vi "Find Exact Peak.vi"(0 "window":T1(ring)=enum."7 Term B-Harris", 1 "Freq. Resolution":dbl=1e-08 format="%0.2e", 2 "Size of FFT (N)":i32=1024 min=0 step=1, 3 "A0":dbl=3.738613052908998e-10 format="%0.8f", 4 "A1":dbl=3.686220325397741e-10 format="%0.8f") -> (5 "A exact":dbl=3.926212591970866e-10 format="%0.8f", 6 "f exact":dbl format="%0.8f")   [LabVIEW 2017, in "NI_AALPro.lvlib"]
doc: "Finds an accurate approximation to the peak response and frequency location using the window coefficients and a binary search algorithm. The best guess is initialized to the center of the frequency bins and is moved within the search loop until the window responses at the bin edges closely approximate the observed magnitude responses of the original spectrum."
uses:
  <vilib>/Analysis/NI_AALPro.lvlib
panel:
  in  "max iterations":i32=100 min=0 step=1
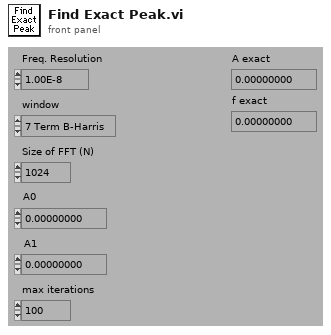
[diagram p1: front panel]
types:
  T1 = enum32{"None ", "Hanning", "Hamming", "Blackman-Harris", "Exact Blackman", "Blackman", "Flat Top", "4 Term B-Harris ", "7 Term B-Harris"}
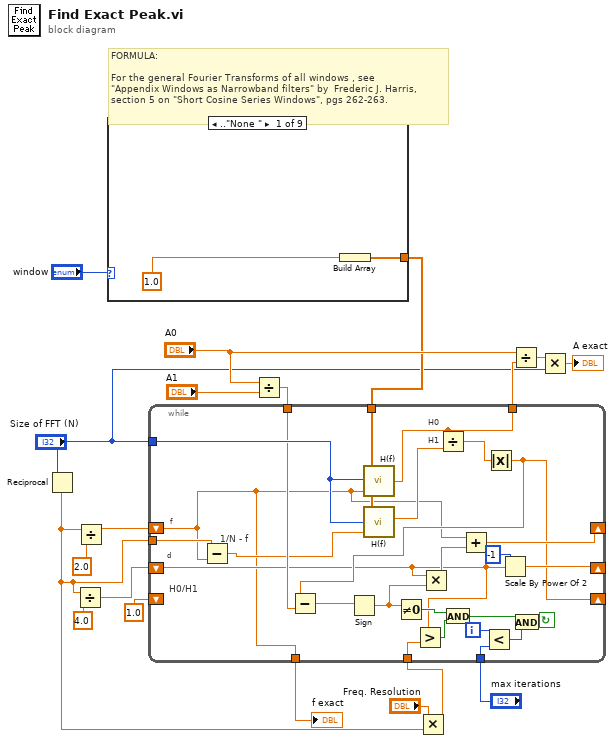
[diagram p0: block diagram]
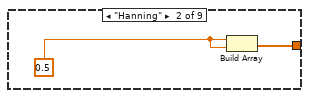
[diagram p2: hidden frame]
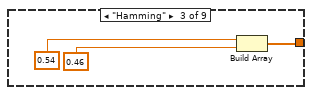
[diagram p3: hidden frame]
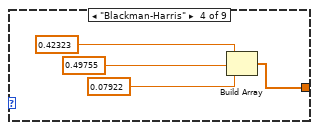
[diagram p4: hidden frame]
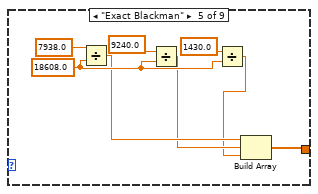
[diagram p5: hidden frame]
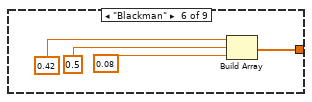
[diagram p6: hidden frame]
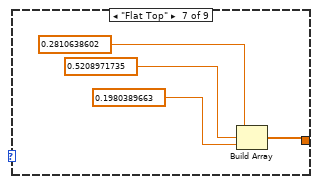
[diagram p7: hidden frame]
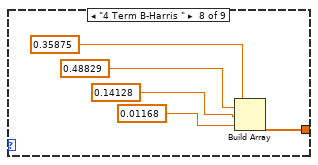
[diagram p8: hidden frame]
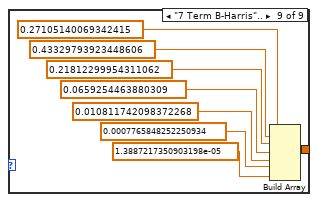
[diagram p9: hidden frame]
diagram:
  # "FORMULA: \n\nFor the general Fourier Transforms of all windows , see \n\"Appendix Windows as Narrowband filters\" by  Frederic J. Harris,\nsection 5 on \"Short Cosine Series Windows\", pgs 262-263."
  n1 = Reciprocal(x="Size of FFT (N)") -> (1/x=w4:dbl)
  n2 = Divide(x=w4, y=4.0) -> (x/y=w14:dbl)
  n3 = Divide(x=w4, y=2.0) -> (x/y=w16:dbl)
  n4 = case shown="..\"None \"" "window" {
    tunnel: [w20 w23 w24 w27 w34 w39 w43 w47 w52] -> w5
    frame .."None " {
      n5 = Build Array(1.0) -> (w20:dbl[])
    }
    frame "Hanning" {
      w22 = 0.5
      n6 = Build Array(w22, w22) -> (w23:dbl[])
    }
    frame "Hamming" {
      n7 = Build Array(0.54, 0.46) -> (w24:dbl[])
    }
    frame "Blackman-Harris" {
      n8 = Build Array(0.42323, 0.49755, 0.07922) -> (w27:dbl[])
    }
    frame "Exact Blackman" {
      w37 = 18608.0
      n9 = Divide(x=7938.0, y=w37) -> (x/y=w33:dbl)
      n10 = Divide(x=9240.0, y=w37) -> (x/y=w32:dbl)
      n11 = Divide(x=1430.0, y=w37) -> (x/y=w31:dbl)
      n12 = Build Array(w33, w32, w31) -> (w34:dbl[])
    }
    frame "Blackman" {
      n13 = Build Array(0.42, 0.5, 0.08) -> (w39:dbl[])
    }
    frame "Flat Top" {
      n14 = Build Array(0.2810638602, 0.5208971735, 0.1980389663) -> (w43:dbl[])
    }
    frame "4 Term B-Harris " {
      n15 = Build Array(0.35875, 0.48829, 0.14128, 0.01168) -> (w47:dbl[])
    }
    frame "7 Term B-Harris".. {
      n16 = Build Array(0.27105140069342415, 0.43329793923448606, 0.21812299954311062, 0.0659254463880309, 0.010811742098372268, 0.0007765848252250934, 1.3887217350903198e-05) -> (w52:dbl[])
    }
  }
  n17 = Divide(x="A0", y="A1") -> (x/y=w7:dbl)
  n18 = Multiply(x="Freq. Resolution", y=w4) -> (x*y=w2:dbl)
  n19 = while {
    tunnel: "max iterations" -> [w64]
    tunnel: w2 -> [w66]
    tunnel: [w62] -> w11
    tunnel: [w60] -> w10
    tunnel: w7 -> [w80]
    shift-left: 1.0 -> [_]
    shift-right: [w73] -> _
    tunnel: w4 -> [w83]
    shift-left: w14 -> [w65]
    shift-right: [w74] -> _
    shift-left: w16 -> [w60]
    shift-right: [w76] -> _
    tunnel: w5 -> [w63]
    tunnel: "Size of FFT (N)" -> [w82]
    i -> [w72]
    stop <- w68 continue-if-true
    # "H0/H1"
    # "d"
    # "1/N - f"
    # "f"
    # "H1"
    # "H0"
    n20 = Subtract(x=w83, y=w60) -> (x-y=w61:dbl)
    n21 = call <vilib>:"H(f).vi"("f"=w60, "N"=w82, "An"=w63) -> ("y"=w62:dbl)
    n22 = call <vilib>:"H(f).vi"("f"=w61, "N"=w82, "An"=w63) -> ("y"=w84:dbl)
    n23 = Greater?(x=w65, y=w66) -> (0:w71:bool)
    n24 = Divide(x=w62, y=w84) -> (x/y=w81:dbl)
    n25 = Less?(x=w72, y=w64) -> (x < y?=w70:bool)
    n26 = Absolute Value(x=w81) -> (abs(x)=w73:dbl)
    n27 = Subtract(x=w73, y=w80) -> (x-y=w67:dbl)
    n28 = Sign(1:w67) -> (0:w78:dbl)
    n29 = Not Equal To 0?(x=w78) -> (x != 0?=w79:bool)
    n30 = Multiply(x=w65, y=w78) -> (x*y=w77:dbl)
    n31 = And(x=w79, y=w71) -> (x .and. y?=w69:bool)
    n32 = Add(x=w60, y=w77) -> (x+y=w76:dbl)
    n33 = Scale By Power Of 2(n=-1, x=w65) -> (x*2^n=w74:dbl)
    n34 = And(x=w69, y=w70) -> (x .and. y?=w68:bool)
  }
  "f exact" <- w10
  n35 = Divide(x="A0", y=w11) -> (x/y=w9:dbl)
  n36 = Multiply(x=w9, y="Size of FFT (N)") -> (x*y=→"A exact":dbl)
